vi "Convert_MPU6050.vi"(1 "Accel Sensor Reading":dbl) -> (0 "Load Force":dbl)   [LabVIEW 2020]
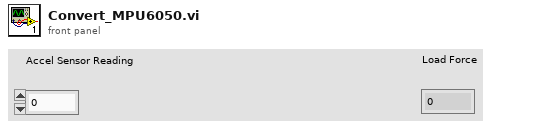
[diagram p1: front panel]
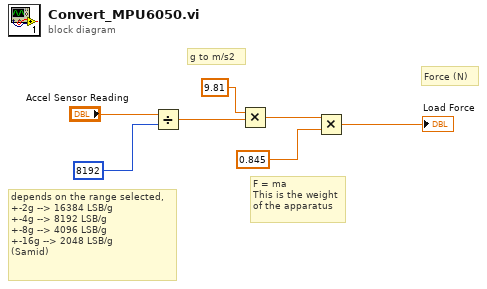
[diagram p0: block diagram]
diagram:
  # "g to m/s2"
  # "depends on the range selected,\n+-2g --> 16384 LSB/g\n+-4g --> 8192 LSB/g\n+-8g --> 4096 LSB/g\n+-16g --> 2048 LSB/g\n(Samid)"
  # "F = ma\nThis is the weight\nof the apparatus"
  # "Force (N)"
  n1 = Divide(x="Accel Sensor Reading", y=8192) -> (x/y=w3:dbl)
  n2 = Multiply(x=9.81 ("y"), y=w3) -> (x*y=w1:dbl)
  n3 = Multiply(x=w1, y=0.845) -> (x*y=→"Load Force":dbl)
